vi "First_Program.vi"(8 "Numeric 3":u8, 9 "Numeric 2":u8, 10 "Numeric":u8) -> ()   [LabVIEW 2015]
panel:
  out "Numeric 4":u8
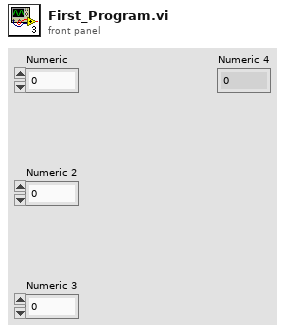
[diagram p1: front panel]
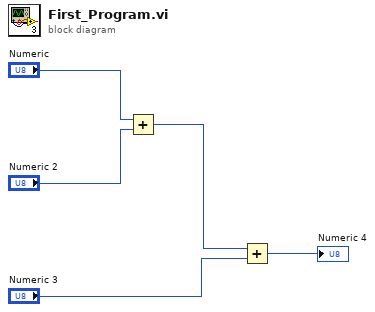
[diagram p0: block diagram]
diagram:
  n1 = Add(x="Numeric", y="Numeric 2") -> (x+y=w1:u8)
  n2 = Add(x=w1, y="Numeric 3") -> (x+y=→"Numeric 4":u8)
